vi "visa mtcdt comm.vi"() -> ()   [LabVIEW 2024]
panel:
  out "return count":u32
  out "error out":errorcluster
  out "read buffer":string
  in  "error in (no error)":errorcluster
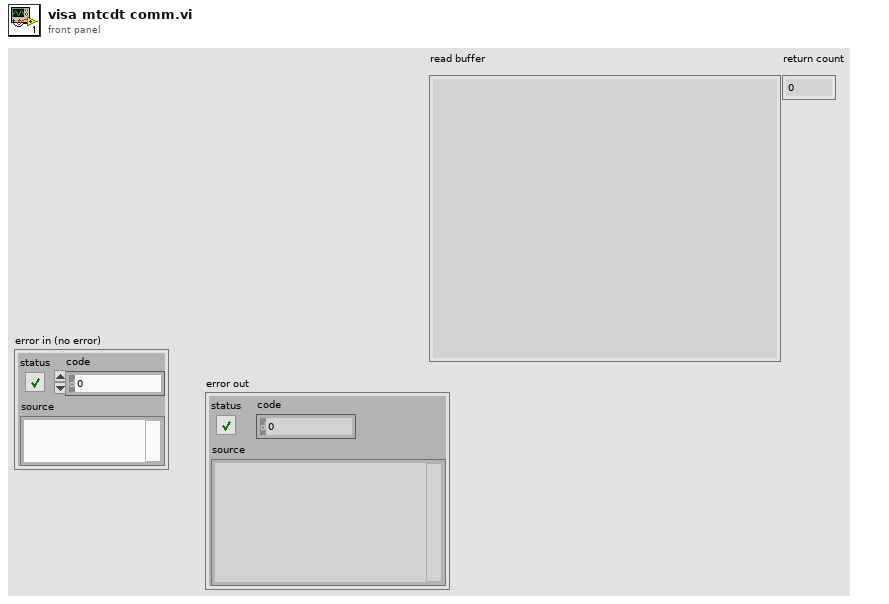
[diagram p1: front panel]
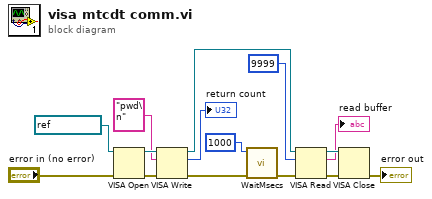
[diagram p0: block diagram]
diagram:
  n1 = VISA Open(error in (no error)="error in (no error)", VISA resource name=refnum<visa-resource-name> "MTCDT") -> (VISA resource name=w13:refnum<visa-resource-name>, error out=w12:errorcluster)  [unwired: 3 in]
  n2 = VISA Write(VISA resource name=w13, write buffer="pwd\n", error in (no error)=w12) -> (VISA resource name out=w2:refnum<visa-resource-name>, return count=→"return count":u32, error out=w10:errorcluster)
  n3 = call "WaitMsecs.vi"("error in (no error)"=w10, "Wait Msecs"=u32 1000) -> ("error out"=w3:errorcluster)  [unwired: 9 in]
  n4 = VISA Read(VISA resource name=w2, byte count=u32 9999, error in (no error)=w3) -> (VISA resource name out=w7:refnum<visa-resource-name>, read buffer=→"read buffer":string, error out=w8:errorcluster)  [unwired: 1 out]
  n5 = VISA Close(VISA resource name=w7, error in (no error)=w8) -> (error out=→"error out":errorcluster)
